vi "Field vs  IV and Ic distribution_V4.vi"() -> ()   [LabVIEW 2024]
uses:
  Ramps.ctl
  RT fast data.ctl
  <vilib>/LabVIEW Targets/FPGA/cRIO/shared/nicrio_ModuleControls/nicrio_cRIO-9775_RecordDataRates4ChansRing.ctl
  <vilib>/LabVIEW Targets/FPGA/cRIO/shared/nicrio_ModuleControls/nicrio_BasicConversionTime.ctl
  <vilib>/Utility/file.llb/Write Delimited Spreadsheet (DBL).vi
  cRIO VI parameters.vi
  <resource>/objmgr/ni.dex.rc
  <vilib>/Analysis/NI_AALBase.lvlib
panel:
  in  "Tab Control":T1(tab)
  in  "Contour plot folder":path=path "C:/Users/gyue/Desktop/GA01_202401"
  in  "Name":string="book827"
  in  "Sample Name":string
  in  "Field Rate mT per sec":dbl=0.1 format="%#_13g"
  in  "Field Radius mT":dbl=6.0 format="%#_13g"
  in  "Field step mT":dbl=0.1 format="%#_13g"
  in  "Field Origin mT":dbl=4.0 format="%#_13g"
  in  "Ramp up first T":bool
  in  "Ramp type":string(combo)="Origin is Boundary"
  in  "Field Device Select":string(combo)="Elsa Magnet mT"
  in  "Power dbm":dbl=-135.0 format="%#_13g"
  in  "Field sub select":string(combo)="50mApV"
  in  "Voltage Scale factor":dbl=0.0001
  in  "Current Scale factor":dbl=1.0
  in  "Relative threshold":dbl=0.18 format="%#_13g"
  in  "Zero avg":i32=1000
  in  "Cutoff delay usec":u32
  in  "Wait before trigger us":u32=10000
  in  "Dist Records Num":i32=10000
  in  "IV Record Data Rate":T2=200 items=["20.000 MS/s (NI 9775)"=1, "10.00 MS/s (NI 9775)"=2, "6.667 MS/s (NI 9775)"=3, "5.000 MS/s (NI 9775)"=4, "2.500 MS/s (NI 9775)"=8, "1.667 MS/s (NI 9775)"=12, "1.250 MS/s (NI 9775)"=16, "1.000 MS/s (NI 9775)"=20, "833.333 KS/s (NI 9775)"=24, "714.286 KS/s (NI 9775)"=28, "625.000 KS/s (NI 9775)"=32, "555.556 KS/s (NI 9775)"=36, "500.000 KS/s (NI 9775)"=40, "454.545 KS/s (NI 9775)"=44, "416.667 KS/s (NI 9775)"=48, "384.615 KS/s (NI 9775)"=52, "357.143 KS/s (NI 9775)"=56, "333.333 KS/s (NI 9775)"=60, "312.500 KS/s (NI 9775)"=64, "294.118 KS/s (NI 9775)"=68, "277.778 KS/s (NI 9775)"=72, "263.158 KS/s (NI 9775)"=76, "250.000 KS/s (NI 9775)"=80, "238.095 KS/s (NI 9775)"=84, "227.273 KS/s (NI 9775)"=88, "217.391 KS/s (NI 9775)"=92, "208.333 KS/s (NI 9775)"=96, "200.000 KS/s (NI 9775)"=100, "192.308 KS/s (NI 9775)"=104, "185.185 KS/s (NI 9775)"=108, "178.571 KS/s (NI 9775)"=112, "172.414 KS/s (NI 9775)"=116, "166.667 KS/s (NI 9775)"=120, "161.290 KS/s (NI 9775)"=124, "156.250 KS/s (NI 9775)"=128, "151.515 KS/s (NI 9775)"=132, "147.059 KS/s (NI 9775)"=136, "142.857 KS/s (NI 9775)"=140, "138.889 KS/s (NI 9775)"=144, "135.135 KS/s (NI 9775)"=148, "131.579 KS/s (NI 9775)"=152, "128.205 KS/s (NI 9775)"=156, "125.000 KS/s (NI 9775)"=160, "121.951 KS/s (NI 9775)"=164, "119.048 KS/s (NI 9775)"=168, "116.279 KS/s (NI 9775)"=172, "113.636 KS/s (NI 9775)"=176, "111.111 KS/s (NI 9775)"=180, "108.696 KS/s (NI 9775)"=184, "106.383 KS/s (NI 9775)"=188, "104.167 KS/s (NI 9775)"=192, "102.041 KS/s (NI 9775)"=196, "100.000 KS/s (NI 9775)"=200, "50.000 KS/s (NI 9775)"=400, "33.333 KS/s (NI 9775)"=600, "25.000 KS/s (NI 9775)"=800, "20.000 KS/s (NI 9775)"=1000, "16.667 KS/s (NI 9775)"=1200, "14.286 KS/s (NI 9775)"=1400, "12.500 KS/s (NI 9775)"=1600, "11.111 KS/s (NI 9775)"=1800, "10.000 KS/s (NI 9775)"=2000, "9.091 KS/s (NI 9775)"=2200, "8.333 KS/s (NI 9775)"=2400, "7.692 KS/s (NI 9775)"=2600, "7.143 KS/s (NI 9775)"=2800, "6.667 KS/s (NI 9775)"=3000, "6.250 KS/s (NI 9775)"=3200, "5.882 KS/s (NI 9775)"=3400, "5.556 KS/s (NI 9775)"=3600, "5.000 KS/s (NI 9775)"=4000, "4.762 KS/s (NI 9775)"=4200, "4.545 KS/s (NI 9775)"=4400, "4.348 KS/s (NI 9775)"=4600, "4.167 KS/s (NI 9775)"=4800, "4.000 KS/s (NI 9775)"=5000, "3.846 KS/s (NI 9775)"=5200, "3.571 KS/s (NI 9775)"=5600, "3.333 KS/s (NI 9775)"=6000, "3.125 KS/s (NI 9775)"=6400, "2.941 KS/s (NI 9775)"=6800, "2.778 KS/s (NI 9775)"=7200, "2.632 KS/s (NI 9775)"=7600, "2.500 KS/s (NI 9775)"=8000, "2.381 KS/s (NI 9775)"=8400, "2.273 KS/s (NI 9775)"=8800, "2.174 KS/s (NI 9775)"=9200, "2.083 KS/s (NI 9775)"=9600, "2.000 KS/s (NI 9775)"=10000, "1.923 KS/s (NI 9775)"=10400, "1.852 KS/s (NI 9775)"=10800, "1.786 KS/s (NI 9775)"=11200, "1.724 KS/s (NI 9775)"=11600, "1.667 KS/s (NI 9775)"=12000, "1.613 KS/s (NI 9775)"=12400, "1.563 KS/s (NI 9775)"=12800, "1.515 KS/s (NI 9775)"=13200, "1.471 KS/s (NI 9775)"=13600, "1.429 KS/s (NI 9775)"=14000, "1.389 KS/s (NI 9775)"=14400, "1.351 KS/s (NI 9775)"=14800, "1.316 KS/s (NI 9775)"=15200, "1.282 KS/s (NI 9775)"=15600, "1.250 KS/s (NI 9775)"=16000, "1.220 KS/s (NI 9775)"=16400, "1.190 KS/s (NI 9775)"=16800, "1.163 KS/s (NI 9775)"=17200, "1.136 KS/s (NI 9775)"=17600, "1.111 KS/s (NI 9775)"=18000, "1.087 KS/s (NI 9775)"=18400, "1.064 KS/s (NI 9775)"=18800, "1.042 KS/s (NI 9775)"=19200, "1.020 KS/s (NI 9775)"=19600, "1.000 KS/s (NI 9775)"=20000, "0.980 KS/s (NI 9775)"=20400, "0.962 KS/s (NI 9775)"=20800, "0.943 KS/s (NI 9775)"=21200, "0.926 KS/s (NI 9775)"=21600, "0.909 KS/s (NI 9775)"=22000, "0.893 KS/s (NI 9775)"=22400, "0.877 KS/s (NI 9775)"=22800, "0.862 KS/s (NI 9775)"=23200, "0.847 KS/s (NI 9775)"=23600, "0.833 KS/s (NI 9775)"=24000, "0.820 KS/s (NI 9775)"=24400, "0.806 KS/s (NI 9775)"=24800, "0.794 KS/s (NI 9775)"=25200, "0.781 KS/s (NI 9775)"=25600, "0.694 KS/s (NI 9775)"=28800, "0.625 KS/s (NI 9775)"=32000, "0.568 KS/s (NI 9775)"=35200, "0.521 KS/s (NI 9775)"=38400, "0.446 KS/s (NI 9775)"=44800, "0.391 KS/s (NI 9775)"=51200, "0.347 KS/s (NI 9775)"=57600, "0.313 KS/s (NI 9775)"=64000]
  in  "IV Record Samples":u32=2300
  in  "Trigger Slope":enum8{"Positive", "Negative"}(ring)
  out "Ramps Cluster":T3={"Amp"=8.0, "Delay time 10us"=1000, "Ramp1 time 10us"=1000, "Ramp2 time 10us"=200, "Ramp3 time 10us"=100, "End time 10us"=0}
  in  "Amp":dbl=8.0
  in  "Delay time 10us":i32=1000
  in  "Ramp1 time 10us":i32=1000
  in  "Ramp2 time 10us":i32=200
  in  "Ramp3 time 10us":i32=100
  in  "End time 10us":i32
  in  "Tab Control 2":enum32{"IV", "Ic"}(tab)
  out "IV parameters":T4={"Records Num"=1, "AI Trigger Configuration"={"Trigger Slope"=enum."Positive", "Trigger Level"=0.10009765625, "Hystesis Value"=0.094970703125, "AI Channel"=0}, "Record PreTrigger Samples"=1, "Record Samples"=2300, "Ic Cut off or curve"=FALSE, "Record Data Rate"=200, "Wait before trigger us"=0, "Cutoff delay usec"=0, "Timing Mode"=enum."High Resolution", "Trigger length ticks"=1, "Timeout"=-1, "Ramps"={"Amp"=8.0, "Delay time 10us"=1000, "Ramp1 time 10us"=1000, "Ramp2 time 10us"=200, "Ramp3 time 10us"=100, "End time 10us"=0}} {"Record Data Rate" items=["20.000 MS/s (NI 9775)"=1, "10.00 MS/s (NI 9775)"=2, "6.667 MS/s (NI 9775)"=3, "5.000 MS/s (NI 9775)"=4, "2.500 MS/s (NI 9775)"=8, "1.667 MS/s (NI 9775)"=12, "1.250 MS/s (NI 9775)"=16, "1.000 MS/s (NI 9775)"=20, "833.333 KS/s (NI 9775)"=24, "714.286 KS/s (NI 9775)"=28, "625.000 KS/s (NI 9775)"=32, "555.556 KS/s (NI 9775)"=36, "500.000 KS/s (NI 9775)"=40, "454.545 KS/s (NI 9775)"=44, "416.667 KS/s (NI 9775)"=48, "384.615 KS/s (NI 9775)"=52, "357.143 KS/s (NI 9775)"=56, "333.333 KS/s (NI 9775)"=60, "312.500 KS/s (NI 9775)"=64, "294.118 KS/s (NI 9775)"=68, "277.778 KS/s (NI 9775)"=72, "263.158 KS/s (NI 9775)"=76, "250.000 KS/s (NI 9775)"=80, "238.095 KS/s (NI 9775)"=84, "227.273 KS/s (NI 9775)"=88, "217.391 KS/s (NI 9775)"=92, "208.333 KS/s (NI 9775)"=96, "200.000 KS/s (NI 9775)"=100, "192.308 KS/s (NI 9775)"=104, "185.185 KS/s (NI 9775)"=108, "178.571 KS/s (NI 9775)"=112, "172.414 KS/s (NI 9775)"=116, "166.667 KS/s (NI 9775)"=120, "161.290 KS/s (NI 9775)"=124, "156.250 KS/s (NI 9775)"=128, "151.515 KS/s (NI 9775)"=132, "147.059 KS/s (NI 9775)"=136, "142.857 KS/s (NI 9775)"=140, "138.889 KS/s (NI 9775)"=144, "135.135 KS/s (NI 9775)"=148, "131.579 KS/s (NI 9775)"=152, "128.205 KS/s (NI 9775)"=156, "125.000 KS/s (NI 9775)"=160, "121.951 KS/s (NI 9775)"=164, "119.048 KS/s (NI 9775)"=168, "116.279 KS/s (NI 9775)"=172, "113.636 KS/s (NI 9775)"=176, "111.111 KS/s (NI 9775)"=180, "108.696 KS/s (NI 9775)"=184, "106.383 KS/s (NI 9775)"=188, "104.167 KS/s (NI 9775)"=192, "102.041 KS/s (NI 9775)"=196, "100.000 KS/s (NI 9775)"=200, "50.000 KS/s (NI 9775)"=400, "33.333 KS/s (NI 9775)"=600, "25.000 KS/s (NI 9775)"=800, "20.000 KS/s (NI 9775)"=1000, "16.667 KS/s (NI 9775)"=1200, "14.286 KS/s (NI 9775)"=1400, "12.500 KS/s (NI 9775)"=1600, "11.111 KS/s (NI 9775)"=1800, "10.000 KS/s (NI 9775)"=2000, "9.091 KS/s (NI 9775)"=2200, "8.333 KS/s (NI 9775)"=2400, "7.692 KS/s (NI 9775)"=2600, "7.143 KS/s (NI 9775)"=2800, "6.667 KS/s (NI 9775)"=3000, "6.250 KS/s (NI 9775)"=3200, "5.882 KS/s (NI 9775)"=3400, "5.556 KS/s (NI 9775)"=3600, "5.000 KS/s (NI 9775)"=4000, "4.762 KS/s (NI 9775)"=4200, "4.545 KS/s (NI 9775)"=4400, "4.348 KS/s (NI 9775)"=4600, "4.167 KS/s (NI 9775)"=4800, "4.000 KS/s (NI 9775)"=5000, "3.846 KS/s (NI 9775)"=5200, "3.571 KS/s (NI 9775)"=5600, "3.333 KS/s (NI 9775)"=6000, "3.125 KS/s (NI 9775)"=6400, "2.941 KS/s (NI 9775)"=6800, "2.778 KS/s (NI 9775)"=7200, "2.632 KS/s (NI 9775)"=7600, "2.500 KS/s (NI 9775)"=8000, "2.381 KS/s (NI 9775)"=8400, "2.273 KS/s (NI 9775)"=8800, "2.174 KS/s (NI 9775)"=9200, "2.083 KS/s (NI 9775)"=9600, "2.000 KS/s (NI 9775)"=10000, "1.923 KS/s (NI 9775)"=10400, "1.852 KS/s (NI 9775)"=10800, "1.786 KS/s (NI 9775)"=11200, "1.724 KS/s (NI 9775)"=11600, "1.667 KS/s (NI 9775)"=12000, "1.613 KS/s (NI 9775)"=12400, "1.563 KS/s (NI 9775)"=12800, "1.515 KS/s (NI 9775)"=13200, "1.471 KS/s (NI 9775)"=13600, "1.429 KS/s (NI 9775)"=14000, "1.389 KS/s (NI 9775)"=14400, "1.351 KS/s (NI 9775)"=14800, "1.316 KS/s (NI 9775)"=15200, "1.282 KS/s (NI 9775)"=15600, "1.250 KS/s (NI 9775)"=16000, "1.220 KS/s (NI 9775)"=16400, "1.190 KS/s (NI 9775)"=16800, "1.163 KS/s (NI 9775)"=17200, "1.136 KS/s (NI 9775)"=17600, "1.111 KS/s (NI 9775)"=18000, "1.087 KS/s (NI 9775)"=18400, "1.064 KS/s (NI 9775)"=18800, "1.042 KS/s (NI 9775)"=19200, "1.020 KS/s (NI 9775)"=19600, "1.000 KS/s (NI 9775)"=20000, "0.980 KS/s (NI 9775)"=20400, "0.962 KS/s (NI 9775)"=20800, "0.943 KS/s (NI 9775)"=21200, "0.926 KS/s (NI 9775)"=21600, "0.909 KS/s (NI 9775)"=22000, "0.893 KS/s (NI 9775)"=22400, "0.877 KS/s (NI 9775)"=22800, "0.862 KS/s (NI 9775)"=23200, "0.847 KS/s (NI 9775)"=23600, "0.833 KS/s (NI 9775)"=24000, "0.820 KS/s (NI 9775)"=24400, "0.806 KS/s (NI 9775)"=24800, "0.794 KS/s (NI 9775)"=25200, "0.781 KS/s (NI 9775)"=25600, "0.694 KS/s (NI 9775)"=28800, "0.625 KS/s (NI 9775)"=32000, "0.568 KS/s (NI 9775)"=35200, "0.521 KS/s (NI 9775)"=38400, "0.446 KS/s (NI 9775)"=44800, "0.391 KS/s (NI 9775)"=51200, "0.347 KS/s (NI 9775)"=57600, "0.313 KS/s (NI 9775)"=64000]}
  out "Ic parameters":T4={"Records Num"=10000, "AI Trigger Configuration"={"Trigger Slope"=enum."Positive", "Trigger Level"=0.2080078125, "Hystesis Value"=0.0, "AI Channel"=0}, "Record PreTrigger Samples"=1, "Record Samples"=16, "Ic Cut off or curve"=TRUE, "Record Data Rate"=1, "Wait before trigger us"=10000, "Cutoff delay usec"=0, "Timing Mode"=enum."High Resolution", "Trigger length ticks"=1, "Timeout"=-1, "Ramps"={"Amp"=8.0, "Delay time 10us"=1000, "Ramp1 time 10us"=1000, "Ramp2 time 10us"=200, "Ramp3 time 10us"=100, "End time 10us"=0}} {"Record Data Rate" items=["20.000 MS/s (NI 9775)"=1, "10.00 MS/s (NI 9775)"=2, "6.667 MS/s (NI 9775)"=3, "5.000 MS/s (NI 9775)"=4, "2.500 MS/s (NI 9775)"=8, "1.667 MS/s (NI 9775)"=12, "1.250 MS/s (NI 9775)"=16, "1.000 MS/s (NI 9775)"=20, "833.333 KS/s (NI 9775)"=24, "714.286 KS/s (NI 9775)"=28, "625.000 KS/s (NI 9775)"=32, "555.556 KS/s (NI 9775)"=36, "500.000 KS/s (NI 9775)"=40, "454.545 KS/s (NI 9775)"=44, "416.667 KS/s (NI 9775)"=48, "384.615 KS/s (NI 9775)"=52, "357.143 KS/s (NI 9775)"=56, "333.333 KS/s (NI 9775)"=60, "312.500 KS/s (NI 9775)"=64, "294.118 KS/s (NI 9775)"=68, "277.778 KS/s (NI 9775)"=72, "263.158 KS/s (NI 9775)"=76, "250.000 KS/s (NI 9775)"=80, "238.095 KS/s (NI 9775)"=84, "227.273 KS/s (NI 9775)"=88, "217.391 KS/s (NI 9775)"=92, "208.333 KS/s (NI 9775)"=96, "200.000 KS/s (NI 9775)"=100, "192.308 KS/s (NI 9775)"=104, "185.185 KS/s (NI 9775)"=108, "178.571 KS/s (NI 9775)"=112, "172.414 KS/s (NI 9775)"=116, "166.667 KS/s (NI 9775)"=120, "161.290 KS/s (NI 9775)"=124, "156.250 KS/s (NI 9775)"=128, "151.515 KS/s (NI 9775)"=132, "147.059 KS/s (NI 9775)"=136, "142.857 KS/s (NI 9775)"=140, "138.889 KS/s (NI 9775)"=144, "135.135 KS/s (NI 9775)"=148, "131.579 KS/s (NI 9775)"=152, "128.205 KS/s (NI 9775)"=156, "125.000 KS/s (NI 9775)"=160, "121.951 KS/s (NI 9775)"=164, "119.048 KS/s (NI 9775)"=168, "116.279 KS/s (NI 9775)"=172, "113.636 KS/s (NI 9775)"=176, "111.111 KS/s (NI 9775)"=180, "108.696 KS/s (NI 9775)"=184, "106.383 KS/s (NI 9775)"=188, "104.167 KS/s (NI 9775)"=192, "102.041 KS/s (NI 9775)"=196, "100.000 KS/s (NI 9775)"=200, "50.000 KS/s (NI 9775)"=400, "33.333 KS/s (NI 9775)"=600, "25.000 KS/s (NI 9775)"=800, "20.000 KS/s (NI 9775)"=1000, "16.667 KS/s (NI 9775)"=1200, "14.286 KS/s (NI 9775)"=1400, "12.500 KS/s (NI 9775)"=1600, "11.111 KS/s (NI 9775)"=1800, "10.000 KS/s (NI 9775)"=2000, "9.091 KS/s (NI 9775)"=2200, "8.333 KS/s (NI 9775)"=2400, "7.692 KS/s (NI 9775)"=2600, "7.143 KS/s (NI 9775)"=2800, "6.667 KS/s (NI 9775)"=3000, "6.250 KS/s (NI 9775)"=3200, "5.882 KS/s (NI 9775)"=3400, "5.556 KS/s (NI 9775)"=3600, "5.000 KS/s (NI 9775)"=4000, "4.762 KS/s (NI 9775)"=4200, "4.545 KS/s (NI 9775)"=4400, "4.348 KS/s (NI 9775)"=4600, "4.167 KS/s (NI 9775)"=4800, "4.000 KS/s (NI 9775)"=5000, "3.846 KS/s (NI 9775)"=5200, "3.571 KS/s (NI 9775)"=5600, "3.333 KS/s (NI 9775)"=6000, "3.125 KS/s (NI 9775)"=6400, "2.941 KS/s (NI 9775)"=6800, "2.778 KS/s (NI 9775)"=7200, "2.632 KS/s (NI 9775)"=7600, "2.500 KS/s (NI 9775)"=8000, "2.381 KS/s (NI 9775)"=8400, "2.273 KS/s (NI 9775)"=8800, "2.174 KS/s (NI 9775)"=9200, "2.083 KS/s (NI 9775)"=9600, "2.000 KS/s (NI 9775)"=10000, "1.923 KS/s (NI 9775)"=10400, "1.852 KS/s (NI 9775)"=10800, "1.786 KS/s (NI 9775)"=11200, "1.724 KS/s (NI 9775)"=11600, "1.667 KS/s (NI 9775)"=12000, "1.613 KS/s (NI 9775)"=12400, "1.563 KS/s (NI 9775)"=12800, "1.515 KS/s (NI 9775)"=13200, "1.471 KS/s (NI 9775)"=13600, "1.429 KS/s (NI 9775)"=14000, "1.389 KS/s (NI 9775)"=14400, "1.351 KS/s (NI 9775)"=14800, "1.316 KS/s (NI 9775)"=15200, "1.282 KS/s (NI 9775)"=15600, "1.250 KS/s (NI 9775)"=16000, "1.220 KS/s (NI 9775)"=16400, "1.190 KS/s (NI 9775)"=16800, "1.163 KS/s (NI 9775)"=17200, "1.136 KS/s (NI 9775)"=17600, "1.111 KS/s (NI 9775)"=18000, "1.087 KS/s (NI 9775)"=18400, "1.064 KS/s (NI 9775)"=18800, "1.042 KS/s (NI 9775)"=19200, "1.020 KS/s (NI 9775)"=19600, "1.000 KS/s (NI 9775)"=20000, "0.980 KS/s (NI 9775)"=20400, "0.962 KS/s (NI 9775)"=20800, "0.943 KS/s (NI 9775)"=21200, "0.926 KS/s (NI 9775)"=21600, "0.909 KS/s (NI 9775)"=22000, "0.893 KS/s (NI 9775)"=22400, "0.877 KS/s (NI 9775)"=22800, "0.862 KS/s (NI 9775)"=23200, "0.847 KS/s (NI 9775)"=23600, "0.833 KS/s (NI 9775)"=24000, "0.820 KS/s (NI 9775)"=24400, "0.806 KS/s (NI 9775)"=24800, "0.794 KS/s (NI 9775)"=25200, "0.781 KS/s (NI 9775)"=25600, "0.694 KS/s (NI 9775)"=28800, "0.625 KS/s (NI 9775)"=32000, "0.568 KS/s (NI 9775)"=35200, "0.521 KS/s (NI 9775)"=38400, "0.446 KS/s (NI 9775)"=44800, "0.391 KS/s (NI 9775)"=51200, "0.347 KS/s (NI 9775)"=57600, "0.313 KS/s (NI 9775)"=64000]}
  out "DAQ_CMD_Writer endpoint":refnum<k21>="DAQ_CMD_Writer"
  out "DAQ_AI_Reader endpoint":refnum<k21>="DAQ_AI_Reader"
  out "PCreaderI":refnum<k21>="PCreaderI"
  out "PC para writer":refnum<k21>="PCwriter"
  out "PCreaderV":refnum<k21>="PCreaderV"
  out "error out":errorcluster
  out "Threshold":dbl=0.207936767578125
  in  "Stop loop":bool
  out "Current Field mT":dbl=3.9000000000000004
  out "Histogram Graph":T6(graph)={"X Values"=[-0.0907666015625, -0.0735693359375, -0.056372070312499994, -0.039174804687499995, -0.021977539062499996, -0.004780273437499996, 0.012416992187500003, 0.029614257812500003, 0.0468115234375, 0.0640087890625, 0.0812060546875, 0.0984033203125, 0.1156005859375, 0.1327978515625, 0.14999511718750003, 0.16719238281250004, 0.18438964843750005, 0.20158691406250007, 0.21878417968750008, 0.2359814453125001, 0.2531787109375001, 0.2703759765625001, 0.28757324218750013, 0.30477050781250015, 0.32196777343750016, 0.3391650390625002, 0.3563623046875002, 0.3735595703125002, 0.3907568359375002, 0.4079541015625002, 0.42515136718750024, 0.44234863281250025, 0.45954589843750027, 0.4767431640625003, 0.4939404296875003, 0.5111376953125003, 0.5283349609375003, 0.5455322265625003, 0.5627294921875003, 0.5799267578125004, 0.5971240234375004, 0.6143212890625004, 0.6315185546875004, 0.6487158203125004, 0.6659130859375004, 0.6831103515625004, 0.7003076171875005, 0.7175048828125005, 0.7347021484375005, 0.7518994140625005, 0.7690966796875005, 0.7862939453125005, 0.8034912109375005, 0.8206884765625005, 0.8378857421875006, 0.8550830078125006, 0.8722802734375006, 0.8894775390625006, 0.9066748046875006, 0.9238720703125006, 0.9410693359375006, 0.9582666015625007, 0.9754638671875007, 0.9926611328125007, 1.0098583984375007, 1.0270556640625006, 1.0442529296875005, 1.0614501953125004, 1.0786474609375003, 1.0958447265625002, 1.1130419921875, 1.1302392578125, 1.1474365234375, 1.1646337890624998, 1.1818310546874997, 1.1990283203124996, 1.2162255859374995, 1.2334228515624994, 1.2506201171874993, 1.2678173828124992, 1.2850146484374991, 1.302211914062499, 1.319409179687499, 1.3366064453124988, 1.3538037109374987, 1.3710009765624986, 1.3881982421874985, 1.4053955078124984, 1.4225927734374983, 1.4397900390624983, 1.4569873046874982, 1.474184570312498, 1.491381835937498, 1.5085791015624979, 1.5257763671874978, 1.5429736328124977, 1.5601708984374976, 1.5773681640624975, 1.5945654296874974, 1.6117626953124973], "Histogram: h(x)"=[1, 0, 0, 0, 0, 0, 0, 0, 0, 0, 0, 0, 0, 0, 0, 0, 0, 0, 0, 0, 0, 0, 0, 0, 0, 0, 0, 0, 0, 0, 0, 0, 0, 0, 0, 0, 0, 0, 0, 0, 0, 0, 0, 0, 0, 0, 0, 0, 0, 1, 4, 2, 8, 11, 16, 27, 46, 62, 80, 116, 141, 196, 223, 306, 318, 391, 412, 382, 538, 523, 555, 490, 592, 539, 524, 536, 457, 459, 382, 358, 276, 239, 202, 149, 136, 81, 66, 52, 40, 29, 17, 8, 2, 3, 2, 1, 0, 0, 0, 1]}
  out "IV curve":cluster{"Y":dbl[], "Y":dbl[]}[](graph)
  # "unit is dBm GHz for RF"
  # "Voltage x factor=uA"
  # "Voltage x factor=V"
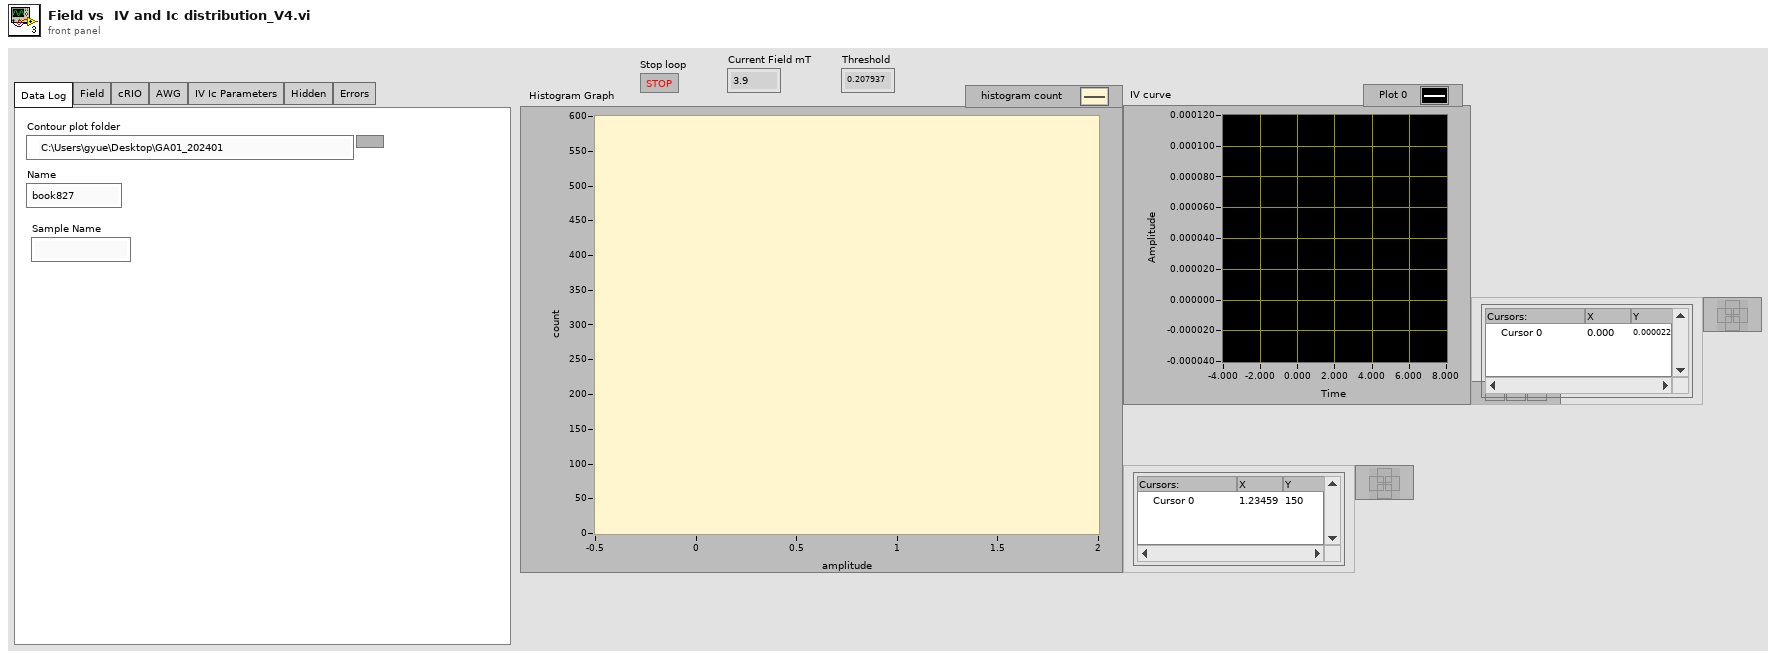
[diagram p1: front panel]
types:
  T1 = enum32{"Data Log", "Field", "cRIO", "AWG", "IV Ic Parameters", "Hidden", "Errors"}
  T2 = typedef "nicrio_cRIO-9775_RecordDataRates4ChansRing.ctl" = u16
  T3 = typedef "Ramps.ctl" = cluster{"Amp":fxp<+/-,20,5>, "Delay time 10us":i32, "Ramp1 time 10us":i32, "Ramp2 time 10us":i32, "Ramp3 time 10us":i32, "End time 10us":i32}
  T4 = typedef "RT fast data.ctl" = cluster{"Records Num":i32, "AI Trigger Configuration":cluster{"Trigger Slope":enum8{"Positive", "Negative"}, "Trigger Level":fxp<+/-,17,5>, "Hystesis Value":fxp<+,16,4>, "AI Channel":u8}, "Record PreTrigger Samples":u32, "Record Samples":u32, "Ic Cut off or curve":bool, "Record Data Rate":T2, "Wait before trigger us":u32, "Cutoff delay usec":u32, "Timing Mode":T5, "Trigger length ticks":u32, "Timeout":i32, "Ramps":T3}
  T5 = typedef "nicrio_BasicConversionTime.ctl" = enum8{"High Speed", "High Resolution"}
  T6 = cluster{"X Values":dbl[], "Histogram: h(x)":i32[]}
  T7 = cluster{"Trigger Slope":enum8{"Positive", "Negative"}, "Trigger Level":fxp<+/-,17,5>, "Hystesis Value":fxp<+,16,4>, "AI Channel":u8}
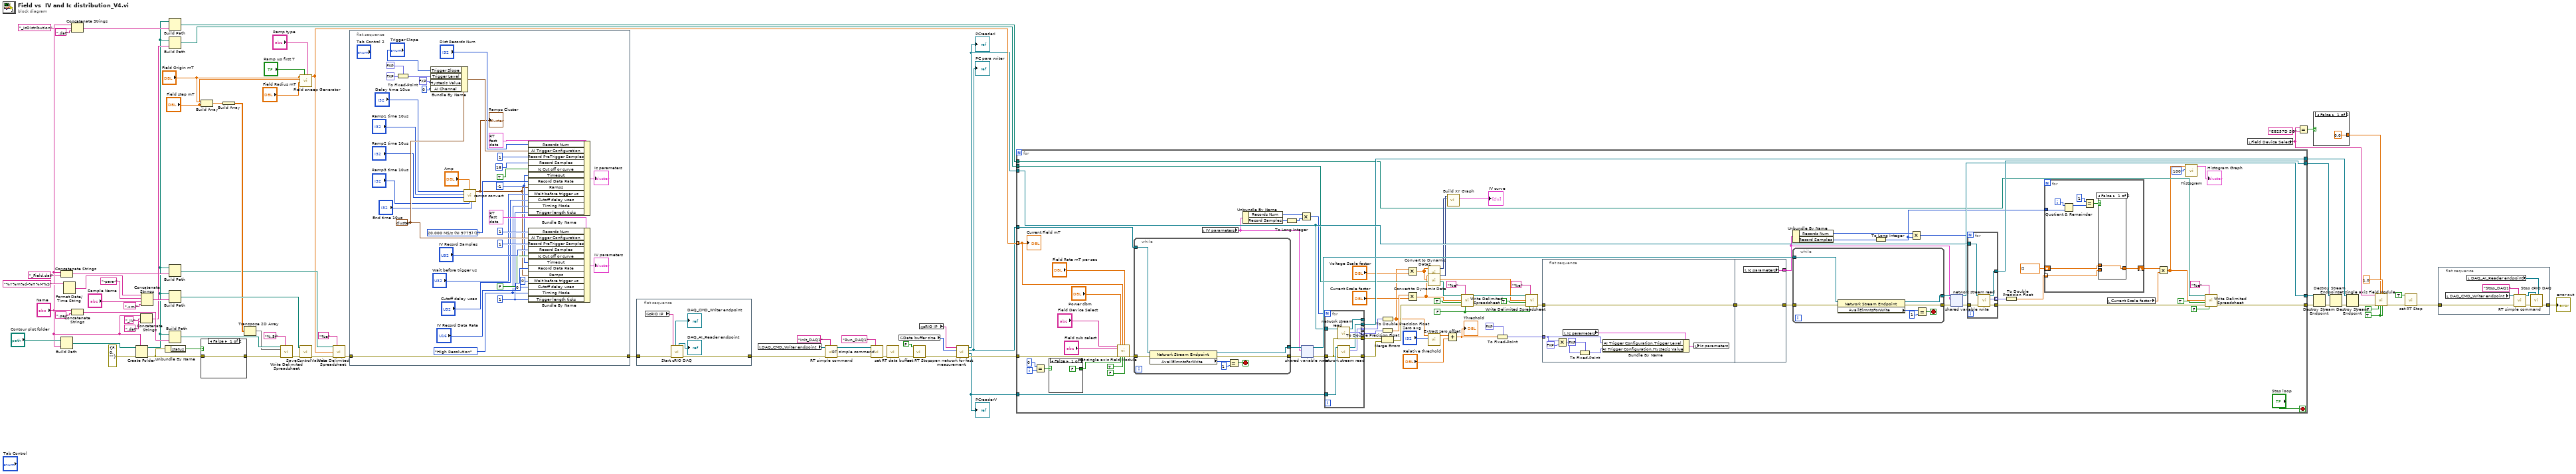
[diagram p0: block diagram]
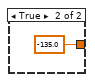
[diagram p2: hidden frame]
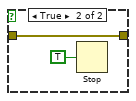
[diagram p3: hidden frame]
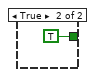
[diagram p4: hidden frame]
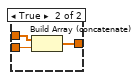
[diagram p5: hidden frame]
diagram:
  w30 = TRUE ("final")
  n1 = Concatenate Strings("Name", "_Field.dat" ("string")) -> (w41:string)
  n2 = Build Path(base path="Contour plot folder", name or relative path="Name") -> (appended path=w58:path)
  n3 = Format Date/Time String(time format string (%c)="%Y%m%d-%H%M%S") -> (date/time string=w54:string)  [unwired: 2 in]
  n4 = Concatenate Strings("Name", "_IcDistribution" ("string"), ".dat" ("string")) -> (w48:string)
  n5 = Concatenate Strings("Name", ".par" ("string")) -> (w65:string)
  n6 = Create Folder(prompt (Create Folder)="Name", path (use dialog)=w58, error in=errorcluster {"status"=FALSE, "code"=0, "source"=""}) -> (created path=w40:path, error out=w55:errorcluster)  [unwired: 1 out]
  n7 = Concatenate Strings("Name", "_IV" ("string"), ".dat" ("string")) -> (w59:string)
  n8 = Concatenate Strings(w54, "-para-" ("string"), "Sample Name", ".xml" ("string")) -> (w69:string)
  n9 = Unbundle By Name(w55) -> ("status"=w56:bool)
  n10 = Build Path(base path=w40, name or relative path=w48) -> (appended path=w46:path)
  n11 = Build Path(base path=w40, name or relative path=w59) -> (appended path=w47:path)
  n12 = Build Path(base path=w40, name or relative path=w41) -> (appended path=w39:path)
  n13 = Build Path(base path=w40, name or relative path=w69) -> (appended path=w67:path)
  n14 = Build Path(base path=w40, name or relative path=w65) -> (appended path=w64:path)
  n15 = Build Array("Field Origin mT", "Field step mT") -> (w62:dbl[])
  n16 = case shown="False" w56 {
    tunnel: [w79 w81] -> w24
    tunnel: w55 -> [w79 w81]
    frame False {
    }
    frame True {
      n17 = Stop(stop? (T)=TRUE) -> ()
    }
  }
  n18 = Build Array(w62) -> (w61:dbl[][])
  n19 = Transpose 2D Array(2D array=w61) -> (transposed array=w60:dbl[][])
  n20 = call-poly <vilib>:"Write Delimited Spreadsheet.vi"("file path (dialog if empty)"=w64, "format (%.3f)"="%.5f", "2D data"=w60, "error in (no error)"=w24) -> ("error out"=w57:errorcluster)  [unwired: 10 in, 1 out]
  n21 = call "Field sweep Generator.vi"("Ramp type"="Ramp type", "Ramp up first T"="Ramp up first T", "Field Radius"="Field Radius mT", "Field step"="Field step mT", "Field Origin"="Field Origin mT") -> ("output array"=w36:dbl[])  [unwired: 6 in]
  n22 = call "SaveControlValues.vi"("XML File Path"=w67, "error in (no error)"=w57) -> ("error out"=w37:errorcluster)  [unwired: 8 in]
  n23 = call-poly <vilib>:"Write Delimited Spreadsheet.vi"("file path (dialog if empty)"=w39, "format (%.3f)"="%e", "1D data"=w36, "error in (no error)"=w37) -> ("error out"=w23:errorcluster)  [unwired: 10 in, 1 out]
  n24 = flat-sequence {
    tunnel: w23 -> [w111]
    tunnel: [w111] -> w17
    frame #0 {
      w91 = -1 ("Timeout")
      w92 = u32 1 ("Trigger length ticks")
      w93 = nicrio_BasicConversionTime."High Resolution" ("Timing Mode")
      w98 = T2 1 items=["20.000 MS/s (NI 9775)"=1, "10.00 MS/s (NI 9775)"=2, "6.667 MS/s (NI 9775)"=3, "5.000 MS/s (NI 9775)"=4, "2.500 MS/s (NI 9775)"=8, "1.667 MS/s (NI 9775)"=12, "1.250 MS/s (NI 9775)"=16, "1.000 MS/s (NI 9775)"=20, "833.333 KS/s (NI 9775)"=24, "714.286 KS/s (NI 9775)"=28, "625.000 KS/s (NI 9775)"=32, "555.556 KS/s (NI 9775)"=36, "500.000 KS/s (NI 9775)"=40, "454.545 KS/s (NI 9775)"=44, "416.667 KS/s (NI 9775)"=48, "384.615 KS/s (NI 9775)"=52, "357.143 KS/s (NI 9775)"=56, "333.333 KS/s (NI 9775)"=60, "312.500 KS/s (NI 9775)"=64, "294.118 KS/s (NI 9775)"=68, "277.778 KS/s (NI 9775)"=72, "263.158 KS/s (NI 9775)"=76, "250.000 KS/s (NI 9775)"=80, "238.095 KS/s (NI 9775)"=84, "227.273 KS/s (NI 9775)"=88, "217.391 KS/s (NI 9775)"=92, "208.333 KS/s (NI 9775)"=96, "200.000 KS/s (NI 9775)"=100, "192.308 KS/s (NI 9775)"=104, "185.185 KS/s (NI 9775)"=108, "178.571 KS/s (NI 9775)"=112, "172.414 KS/s (NI 9775)"=116, "166.667 KS/s (NI 9775)"=120, "161.290 KS/s (NI 9775)"=124, "156.250 KS/s (NI 9775)"=128, "151.515 KS/s (NI 9775)"=132, "147.059 KS/s (NI 9775)"=136, "142.857 KS/s (NI 9775)"=140, "138.889 KS/s (NI 9775)"=144, "135.135 KS/s (NI 9775)"=148, "131.579 KS/s (NI 9775)"=152, "128.205 KS/s (NI 9775)"=156, "125.000 KS/s (NI 9775)"=160, "121.951 KS/s (NI 9775)"=164, "119.048 KS/s (NI 9775)"=168, "116.279 KS/s (NI 9775)"=172, "113.636 KS/s (NI 9775)"=176, "111.111 KS/s (NI 9775)"=180, "108.696 KS/s (NI 9775)"=184, "106.383 KS/s (NI 9775)"=188, "104.167 KS/s (NI 9775)"=192, "102.041 KS/s (NI 9775)"=196, "100.000 KS/s (NI 9775)"=200, "50.000 KS/s (NI 9775)"=400, "33.333 KS/s (NI 9775)"=600, "25.000 KS/s (NI 9775)"=800, "20.000 KS/s (NI 9775)"=1000, "16.667 KS/s (NI 9775)"=1200, "14.286 KS/s (NI 9775)"=1400, "12.500 KS/s (NI 9775)"=1600, "11.111 KS/s (NI 9775)"=1800, "10.000 KS/s (NI 9775)"=2000, "9.091 KS/s (NI 9775)"=2200, "8.333 KS/s (NI 9775)"=2400, "7.692 KS/s (NI 9775)"=2600, "7.143 KS/s (NI 9775)"=2800, "6.667 KS/s (NI 9775)"=3000, "6.250 KS/s (NI 9775)"=3200, "5.882 KS/s (NI 9775)"=3400, "5.556 KS/s (NI 9775)"=3600, "5.000 KS/s (NI 9775)"=4000, "4.762 KS/s (NI 9775)"=4200, "4.545 KS/s (NI 9775)"=4400, "4.348 KS/s (NI 9775)"=4600, "4.167 KS/s (NI 9775)"=4800, "4.000 KS/s (NI 9775)"=5000, "3.846 KS/s (NI 9775)"=5200, "3.571 KS/s (NI 9775)"=5600, "3.333 KS/s (NI 9775)"=6000, "3.125 KS/s (NI 9775)"=6400, "2.941 KS/s (NI 9775)"=6800, "2.778 KS/s (NI 9775)"=7200, "2.632 KS/s (NI 9775)"=7600, "2.500 KS/s (NI 9775)"=8000, "2.381 KS/s (NI 9775)"=8400, "2.273 KS/s (NI 9775)"=8800, "2.174 KS/s (NI 9775)"=9200, "2.083 KS/s (NI 9775)"=9600, "2.000 KS/s (NI 9775)"=10000, "1.923 KS/s (NI 9775)"=10400, "1.852 KS/s (NI 9775)"=10800, "1.786 KS/s (NI 9775)"=11200, "1.724 KS/s (NI 9775)"=11600, "1.667 KS/s (NI 9775)"=12000, "1.613 KS/s (NI 9775)"=12400, "1.563 KS/s (NI 9775)"=12800, "1.515 KS/s (NI 9775)"=13200, "1.471 KS/s (NI 9775)"=13600, "1.429 KS/s (NI 9775)"=14000, "1.389 KS/s (NI 9775)"=14400, "1.351 KS/s (NI 9775)"=14800, "1.316 KS/s (NI 9775)"=15200, "1.282 KS/s (NI 9775)"=15600, "1.250 KS/s (NI 9775)"=16000, "1.220 KS/s (NI 9775)"=16400, "1.190 KS/s (NI 9775)"=16800, "1.163 KS/s (NI 9775)"=17200, "1.136 KS/s (NI 9775)"=17600, "1.111 KS/s (NI 9775)"=18000, "1.087 KS/s (NI 9775)"=18400, "1.064 KS/s (NI 9775)"=18800, "1.042 KS/s (NI 9775)"=19200, "1.020 KS/s (NI 9775)"=19600, "1.000 KS/s (NI 9775)"=20000, "0.980 KS/s (NI 9775)"=20400, "0.962 KS/s (NI 9775)"=20800, "0.943 KS/s (NI 9775)"=21200, "0.926 KS/s (NI 9775)"=21600, "0.909 KS/s (NI 9775)"=22000, "0.893 KS/s (NI 9775)"=22400, "0.877 KS/s (NI 9775)"=22800, "0.862 KS/s (NI 9775)"=23200, "0.847 KS/s (NI 9775)"=23600, "0.833 KS/s (NI 9775)"=24000, "0.820 KS/s (NI 9775)"=24400, "0.806 KS/s (NI 9775)"=24800, "0.794 KS/s (NI 9775)"=25200, "0.781 KS/s (NI 9775)"=25600, "0.694 KS/s (NI 9775)"=28800, "0.625 KS/s (NI 9775)"=32000, "0.568 KS/s (NI 9775)"=35200, "0.521 KS/s (NI 9775)"=38400, "0.446 KS/s (NI 9775)"=44800, "0.391 KS/s (NI 9775)"=51200, "0.347 KS/s (NI 9775)"=57600, "0.313 KS/s (NI 9775)"=64000] ("Record Data Rate")
      w106 = T7 {"Trigger Slope"=enum."Positive", "Trigger Level"=0.10009765625, "Hystesis Value"=0.094970703125, "AI Channel"=0} ("AI Trigger Configuration")
      n25 = To Fixed-Point(fixed-point type=fxp<+/-,17,5> 0.0 ("Trigger Level"), number=fxp<+/-,32,16> 0.0) -> (fixed-point=w103:fxp<+/-,17,5>)
      n26 = Bundle By Name(cluster=w106, "Trigger Slope"="Trigger Slope", "Trigger Level"=w103, "Hystesis Value"=fxp<+,16,4> 0.0, "AI Channel"=u8 0) -> (w100:T7)
      n27 = call "ramps convert.vi"("End time 10us"="End time 10us", "Ramp3 time 10us"="Ramp3 time 10us", "Amp"="Amp", "Ramp2 time 10us"="Ramp2 time 10us", "Ramp1 time 10us"="Ramp1 time 10us", "Delay time 10us"="Delay time 10us") -> ("Ramps cluster"=w84:T3)  [unwired: 5 in]
      "Ramps Cluster" <- w84
      n28 = Bundle By Name(cluster=T4 {"Records Num"=1, "AI Trigger Configuration"={"Trigger Slope"=enum."Positive", "Trigger Level"=0.10009765625, "Hystesis Value"=0.094970703125, "AI Channel"=0}, "Record PreTrigger Samples"=1, "Record Samples"=5000, "Ic Cut off or curve"=FALSE, "Record Data Rate"=200, "Wait before trigger us"=10100, "Cutoff delay usec"=500, "Timing Mode"=enum."High Resolution", "Trigger length ticks"=15, "Timeout"=-1, "Ramps"={"Amp"=0.0, "Delay time 10us"=1, "Ramp1 time 10us"=1000, "Ramp2 time 10us"=2000, "Ramp3 time 10us"=1000, "End time 10us"=1}} ("IV parameters 2"), "Records Num"="Dist Records Num", "AI Trigger Configuration"=w100, "Record PreTrigger Samples"=u32 1, "Record Samples"=u32 16, "Ic Cut off or curve"=TRUE, "Timeout"=w91, "Record Data Rate"=w98, "Ramps"=w84, "Wait before trigger us"="Wait before trigger us", "Cutoff delay usec"="Cutoff delay usec", "Timing Mode"=w93, "Trigger length ticks"=w92) -> (→"Ic parameters":T4)
      n29 = Bundle By Name(cluster=T4 {"Records Num"=1, "AI Trigger Configuration"={"Trigger Slope"=enum."Positive", "Trigger Level"=0.10009765625, "Hystesis Value"=0.094970703125, "AI Channel"=0}, "Record PreTrigger Samples"=1, "Record Samples"=5000, "Ic Cut off or curve"=FALSE, "Record Data Rate"=200, "Wait before trigger us"=10100, "Cutoff delay usec"=500, "Timing Mode"=enum."High Resolution", "Trigger length ticks"=15, "Timeout"=-1, "Ramps"={"Amp"=0.0, "Delay time 10us"=1, "Ramp1 time 10us"=1000, "Ramp2 time 10us"=2000, "Ramp3 time 10us"=1000, "End time 10us"=1}} ("IV parameters 2"), "Records Num"=1, "AI Trigger Configuration"=w106, "Record PreTrigger Samples"=u32 1, "Record Samples"="IV Record Samples", "Ic Cut off or curve"=FALSE, "Timeout"=w91, "Record Data Rate"="IV Record Data Rate", "Ramps"=w84, "Wait before trigger us"=u32 0, "Cutoff delay usec"=u32 0, "Timing Mode"=w93, "Trigger length ticks"=w92) -> (→"IV parameters":T4)
    }
  }
  n30 = flat-sequence {
    tunnel: w17 -> [w121]
    tunnel: [w120] -> w16
    frame #0 {
      n31 = global read "cRIO VI parameters.vi" "cRIO IP"() -> (w119:string)
      n32 = call "Start cRIO DAQ.vi"("error in (no error)"=w121, "cRIO IP"=w119) -> ("error out"=w120:errorcluster, "DAQ_AI_Reader endpoint"=→"DAQ_AI_Reader endpoint":refnum<k21>, "DAQ_CMD_Writer endpoint"=→"DAQ_CMD_Writer endpoint":refnum<k21>)  [unwired: 7 in]
    }
  }
  n33 = local read "DAQ_CMD_Writer endpoint"() -> (w22:refnum<k21>)
  n34 = call "RT simple command.vi"("Command"="Init_DAQ1", "error in (no error)"=w16, "DAQ_CMD_Writer endpoint"=w22) -> ("error out"=w20:errorcluster, "DAQ_CMD_Writer endpoint out"=w19:refnum<k21>)  [unwired: 7 in]
  n35 = call "RT simple command.vi"("Command"="Run_DAQ1", "error in (no error)"=w20, "DAQ_CMD_Writer endpoint"=w19) -> ("error out"=w9:errorcluster)  [unwired: 7 in, 1 out]
  n36 = call "set RT data buffer.vi"("error in (no error)"=w9) -> ("error out"=w8:errorcluster)  [unwired: 10 in]
  n37 = global read "cRIO VI parameters.vi" "Data buffer size"() -> (w4:i32)
  n38 = call "set RT Stop.vi"("error in (no error)"=w8, "RT Stop"=FALSE) -> ("error out"=w7:errorcluster)  [unwired: 9 in]
  n39 = global read "cRIO VI parameters.vi" "cRIO IP"() -> (w5:string)
  n40 = call "open network for fast measurement.vi"("error in (no error)"=w7, "Data buffer size"=w4, "cRIO IP"=w5) -> ("error out"=w15:errorcluster, "PCreaderV"=w12:refnum<k21>, "PC para writer"=w14:refnum<k21>, "PCreaderI"=w13:refnum<k21>)  [unwired: 5 in]
  "PCreaderI" <- w13
  "PC para writer" <- w14
  "PCreaderV" <- w12
  n41 = for {
    tunnel: w14 -> [w204]
    tunnel: [w193] -> w75
    tunnel: w15 -> [w141]
    tunnel: [w161] -> w73
    tunnel: w13 -> [w198]
    tunnel: [w196] -> w76
    tunnel: w12 -> [w182]
    tunnel: [w181] -> w74
    tunnel: w47 -> [w167]
    tunnel: w46 -> [w159]
    tunnel: w36 -> [w139] mode=indexing
    i -> [w135]
    stop <- "Stop loop" stop-if-true
    w151 = FALSE ("transpose? (no:F)")
    n42 = Equal?(x=0, y=w135) -> (x = y?=w133:bool)
    n43 = case shown="False" w133 {
      tunnel: [FALSE ("Init") TRUE ("Init")] -> w132
      frame False {
      }
      frame True {
      }
    }
    n44 = call "set single axis Field Module.vi"("Field Device Select"="Field Device Select", "Field sub select"="Field sub select", "error in (no error)"=w141, "Power dbm"="Power dbm", "Init"=w132, "Field Target mT or dBm"=w139, "Exec"=TRUE, "Field Rate mT per sec"="Field Rate mT per sec", "final"=FALSE) -> ("error out"=w140:errorcluster)  [unwired: 10 in]
    n45 = while {
      tunnel: w204 -> [w257]
      tunnel: w140 -> [w256]
      tunnel: [w252] -> w205
      tunnel: [w251] -> w203
      stop <- w253 stop-if-true
      n46 = property class="Network Stream Endpoint"(reference=w257, error in=w256) -> (reference out=w252:refnum<k21>, error out=w251:errorcluster, "AvailElmntsForWrite"=w255:i32)
      n47 = Equal?(x=w255, y=1) -> (x = y?=w253:bool)
    }
    n48 = local read "IV parameters"() -> (w187:T4)
    n49 = Unbundle By Name(w187) -> ("Records Num"=w186:i32, "Record Samples"=w185:u32)
    n50 = To Long Integer(number=w185) -> (32bit integer=w184:i32)
    n51 = Multiply(x=w186, y=w184) -> (x*y=w183:i32)
    n52 = shared-variable-write(w205, w203, w187) -> (w201:refnum<k21>, w202:errorcluster)  [unwired: 1 in, 1 out]
    n53 = for {
      N: w183 -> [_]
      tunnel: w198 -> [w250]
      tunnel: w202 -> [w243]
      tunnel: [w249] -> w166 mode=indexing
      tunnel: [w248] -> _
      tunnel: [w247] -> w180
      tunnel: w182 -> [w246]
      tunnel: [w245] -> w181
      tunnel: [w244] -> w165 mode=indexing
      tunnel: [w242] -> w179
      n54 = call "network stream read.vi"("error in (no error)"=w243, "endpoint in"=w250) -> ("error out"=w247:errorcluster, "Data"=w249:fxp<+/-,17,5>, "endpoint out"=w248:refnum<k21>)  [unwired: 7 in]
      n55 = call "network stream read.vi"("error in (no error)"=w243, "endpoint in"=w246) -> ("error out"=w242:errorcluster, "Data"=w244:fxp<+/-,17,5>, "endpoint out"=w245:refnum<k21>)  [unwired: 7 in]
    }
    n56 = To Double Precision Float(number=w166) -> (double precision float=w150:dbl[])
    n57 = Merge Errors(w180, w179) -> (w172:errorcluster)
    n58 = To Double Precision Float(number=w165) -> (double precision float=w126:dbl[])
    n59 = Multiply(x=w126, y="Voltage Scale factor") -> (x*y=w146:dbl[])
    n60 = Multiply(x=w150, y="Current Scale factor") -> (x*y=w148:dbl[])
    n61 = call "Convert to Dynamic Data2"("Array"=w146) -> ("Dynamic Data Type"=w191:dynamicdata)  [unwired: 3 in]
    n62 = call "Convert to Dynamic Data"("Array"=w148) -> ("Dynamic Data Type"=w192:dynamicdata)  [unwired: 3 in]
    n63 = call "Extract zero offset.vi"("Zero avg num"="Zero avg", "Array"=w126) -> ("Offset"=w124:dbl)  [unwired: 9 in]
    n64 = Add(x=w124, y="Relative threshold") -> (x+y=w142:dbl)
    "Threshold" <- w142
    n65 = call "Build XY Graph"("Y Input"=w191, "X Input"=w192) -> ("XY Graph"=→"IV curve":cluster{"X":dbl[], "Y":dbl[]}[])  [unwired: 8 in, 1 out]
    n66 = call-poly <vilib>:"Write Delimited Spreadsheet.vi"("file path (dialog if empty)"=w167, "format (%.3f)"="%e", "1D data"=w148, "append to file? (new file:F)"=TRUE, "error in (no error)"=w172, "transpose? (no:F)"=w151) -> ("new file path (Not A Path if cancelled)"=w168:path, "error out"=w169:errorcluster)  [unwired: 8 in]
    n67 = To Fixed-Point(fixed-point type=fxp<+,16,4> 0.0 ("AI Trigger Configuration.Hystesis Value"), number=w142) -> (fixed-point=w156:fxp<+,16,4>)
    n68 = call-poly <vilib>:"Write Delimited Spreadsheet.vi"("file path (dialog if empty)"=w168, "format (%.3f)"="%e", "1D data"=w146, "append to file? (new file:F)"=TRUE, "error in (no error)"=w169, "transpose? (no:F)"=w151) -> ("error out"=w154:errorcluster)  [unwired: 8 in, 1 out]
    n69 = flat-sequence {
      tunnel: w156 -> [w212]
      tunnel: w154 -> [w213]
      tunnel: [w213] -> w137
      tunnel: [w217] -> w153
      tunnel: w137 -> [w217]
      tunnel: [w216] -> w136
      frame #0 {
        n70 = Multiply(x=w212, y=fxp<+,16,4> 0.0) -> (x*y=w210:fxp<+,32,8>)
        n71 = local read "Ic parameters"() -> (w215:T4)
        n72 = To Fixed-Point(fixed-point type=fxp<+,16,4> 0.0 ("AI Trigger Configuration.Hystesis Value"), number=w210) -> (fixed-point=w211:fxp<+,16,4>)
        n73 = Bundle By Name(cluster=w215, "AI Trigger Configuration.Trigger Level"=w212, "AI Trigger Configuration.Hystesis Value"=w211) -> (w214:T4)
        n74 = local write "Ic parameters"(w214) -> ()
      }
      frame #1 {
        n75 = local read "Ic parameters"() -> (w216:T4)
      }
    }
    n76 = Unbundle By Name(w136) -> ("Records Num"=w190:i32, "Record Samples"=w189:u32)
    n77 = while {
      tunnel: w201 -> [w239]
      tunnel: w153 -> [w238]
      tunnel: [w236] -> w200
      tunnel: [w235] -> w199
      stop <- w237 stop-if-true
      n78 = property class="Network Stream Endpoint"(reference=w239, error in=w238) -> (reference out=w236:refnum<k21>, error out=w235:errorcluster, "AvailElmntsForWrite"=w241:i32)
      n79 = Equal?(x=w241, y=1) -> (x = y?=w237:bool)
    }
    n80 = To Long Integer(number=w189) -> (32bit integer=w176:i32)
    n81 = Multiply(x=w190, y=w176) -> (x*y=w188:i32)
    n82 = shared-variable-write(w200, w199, w136) -> (w193:refnum<k21>, w197:errorcluster)  [unwired: 1 in, 1 out]
    n83 = for {
      N: w188 -> [_]
      tunnel: w198 -> [w234]
      tunnel: w197 -> [w233]
      tunnel: [w232] -> w162
      tunnel: [w231] -> w196
      tunnel: [w230] -> w194 mode=indexing
      n84 = call "network stream read.vi"("error in (no error)"=w233, "endpoint in"=w234) -> ("error out"=w232:errorcluster, "Data"=w230:fxp<+/-,17,5>, "endpoint out"=w231:refnum<k21>)  [unwired: 7 in]
    }
    n85 = To Double Precision Float(number=w194) -> (double precision float=w160:dbl[])
    n86 = for {
      tunnel: w160 -> [w219] mode=indexing
      tunnel: w176 -> [w225]
      shift-right: [w221] -> w145
      shift-left: dbl[] [] -> [w220]
      i -> [w224]
      n87 = Quotient & Remainder(x=w224, y=w225) -> (x-y*floor(x/y)=w223:i32)  [unwired: 1 out]
      n88 = Equal?(x=1, y=w223) -> (x = y?=w218:bool)
      n89 = case shown="False" w218 {
        tunnel: [w226 w229] -> w221
        tunnel: w220 -> [w226 w228]
        tunnel: w219 -> [_ w227]
        frame False {
        }
        frame True {
          n90 = Build Array (concatenate)(w228, w227) -> (w229:dbl[])
        }
      }
    }
    n91 = local read "Current Scale factor"() -> (w143:dbl)
    n92 = Multiply(x=w145, y=w143) -> (x*y=w144:dbl[])
    n93 = call <vilib>:"Histogram.vi"("intervals"=100, "X"=w144) -> ("Histogram Graph"=→"Histogram Graph":T6)  [unwired: 6 in, 3 out]
    n94 = call-poly <vilib>:"Write Delimited Spreadsheet.vi"("file path (dialog if empty)"=w159, "format (%.3f)"="%e", "1D data"=w144, "append to file? (new file:F)"=TRUE, "error in (no error)"=w162, "transpose? (no:F)"=FALSE) -> ("error out"=w161:errorcluster)  [unwired: 8 in, 1 out]
    "Current Field mT" <- w139
  }
  n95 = local read "Field Device Select"() -> (w28:string)
  n96 = Equal?(x=w28, y="E8257D SG") -> (x = y?=w26:bool)
  n97 = case shown="False" w26 {
    tunnel: [0.0 ("Field Target mT") -135.0 ("Field Target mT")] -> w25
    frame False {
    }
    frame True {
    }
  }
  n98 = Destroy Stream Endpoint(8:w73, 11:w75) -> (0:w78:errorcluster)
  n99 = Destroy Stream Endpoint(8:w78, 11:w76) -> (0:w77:errorcluster)
  n100 = Destroy Stream Endpoint(8:w77, 11:w74) -> (0:w33:errorcluster)
  n101 = call "set single axis Field Module.vi"("Field Device Select"=w28, "error in (no error)"=w33, "Init"=FALSE, "Field Target mT or dBm"=w25, "Exec"=w30, "Field Rate mT per sec"=1.0, "final"=w30) -> ("error out"=w3:errorcluster)  [unwired: 12 in]
  n102 = call "set RT Stop.vi"("error in (no error)"=w3, "RT Stop"=TRUE) -> ("error out"=w2:errorcluster)  [unwired: 9 in]
  n103 = flat-sequence {
    tunnel: w2 -> [w262]
    tunnel: [w260] -> w11
    frame #0 {
      n104 = local read "DAQ_CMD_Writer endpoint"() -> (w263:refnum<k21>)
      n105 = local read "DAQ_AI_Reader endpoint"() -> (w261:refnum<k21>)
      n106 = call "RT simple command.vi"("Command"="Stop_DAQ1", "error in (no error)"=w262, "DAQ_CMD_Writer endpoint"=w263) -> ("error out"=w266:errorcluster, "DAQ_CMD_Writer endpoint out"=w264:refnum<k21>)  [unwired: 7 in]
      n107 = call "Stop cRIO DAQ.vi"("DAQ_AI_Reader endpoint"=w261, "DAQ_CMD_Writer endpoint"=w264, "error in (no error)"=w266) -> ("error out"=w260:errorcluster)  [unwired: 8 in]
    }
  }
  "error out" <- w11
